vi "PatternRecognition.vi"() -> ()   [LabVIEW 2021]
uses:
  <vilib>/Analysis/baseanly.llb/Normalize Matrix.vi
  <vilib>/numeric/Random Number (Range) I64.vi
  <vilib>/Analysis/baseanly.llb/Real A x B.vi
  <vilib>/numeric/sub_Random U32.vi
  <vilib>/Analysis/Matrix/Numeric/Conversions/Matrix To Array - RM.vi
  <vilib>/Analysis/NI_AALBase.lvlib
  <vilib>/Analysis/Matrix/NI_Matrix.lvlib
  <vilib>/vision/NI_Vision_Development_Module.lvlib
panel:
  out "Confidence":dbl
  out "Pattern":dbl
  out "min value":dbl
  out "max value":dbl
  out "Elapsed Time Text":string
  out "Image":T1(plugin-control)
  in  "Init - Random":bool
  in  "index":i32
  in  "Paths":path[](array[path])
  out "Image Pixels":sgl[][](array[numeric])
  in  "Output":i32=1
  in  "2th layer":i32=2
  in  "1th layer":i32=3
  in  "Predict":bool
  out "Error":dbl[](array[numeric])
  in  "W1":dbl[][](array[numeric])
  out "Y":dbl[][](array[numeric])
  in  "Learn?":bool
  in  "Lr":dbl
  in  "stop":bool
  in  "Y_ideal":dbl[][][](array[numeric])
  in  "Bias 2":dbl[][](array[numeric]) format="%#_13g"
  in  "Bias 3":dbl[][](array[numeric]) format="%#_13g"
  in  "Bias 1":dbl[][](array[numeric]) format="%#_13g"
  in  "W2":dbl[][](array[numeric])
  in  "W3":dbl[][](array[numeric])
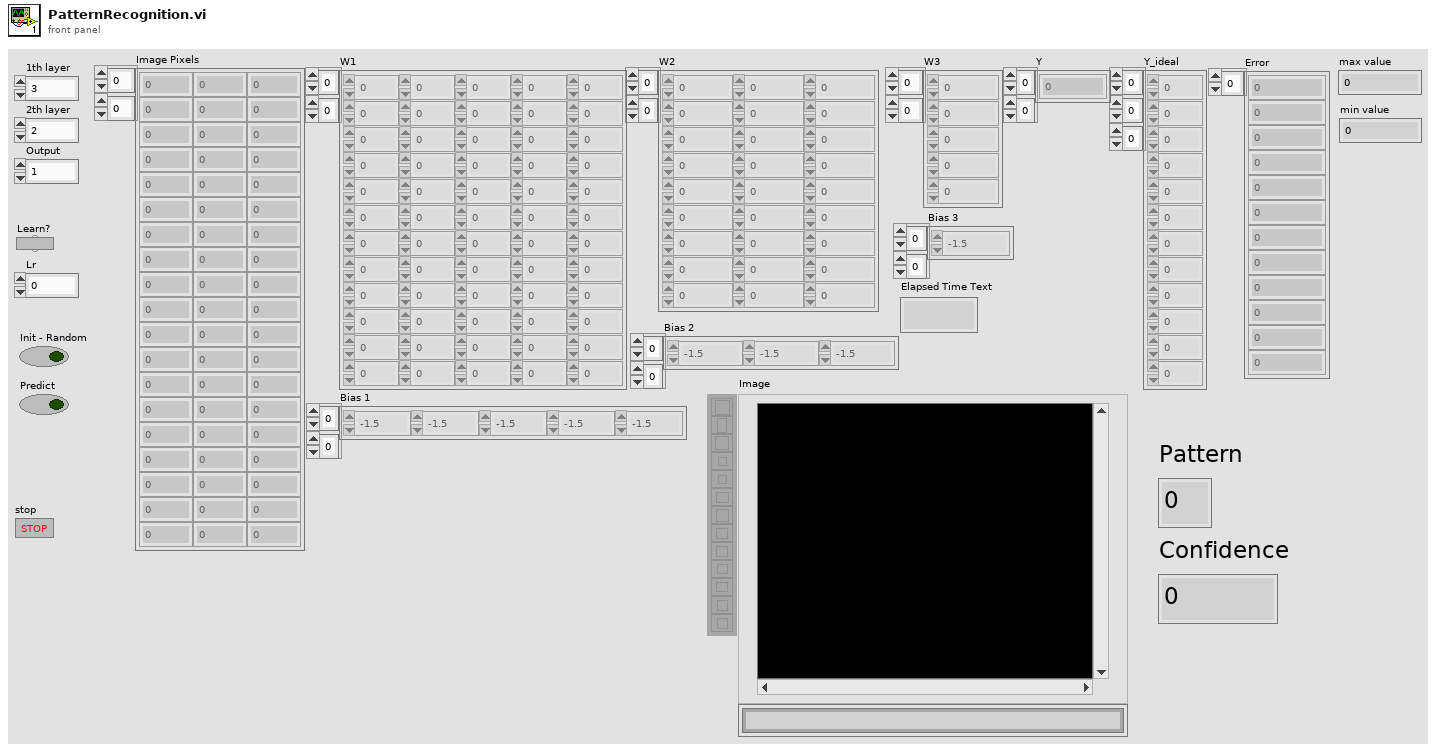
[diagram p1: front panel]
types:
  T1 = typedef "IMAQ Image.ctl" = refnum<image>
  T2 = typedef "Image Type" = u32
  T3 = typedef "NI_Matrix.lvlib/RealMatrix.ctl" = dbl[][]
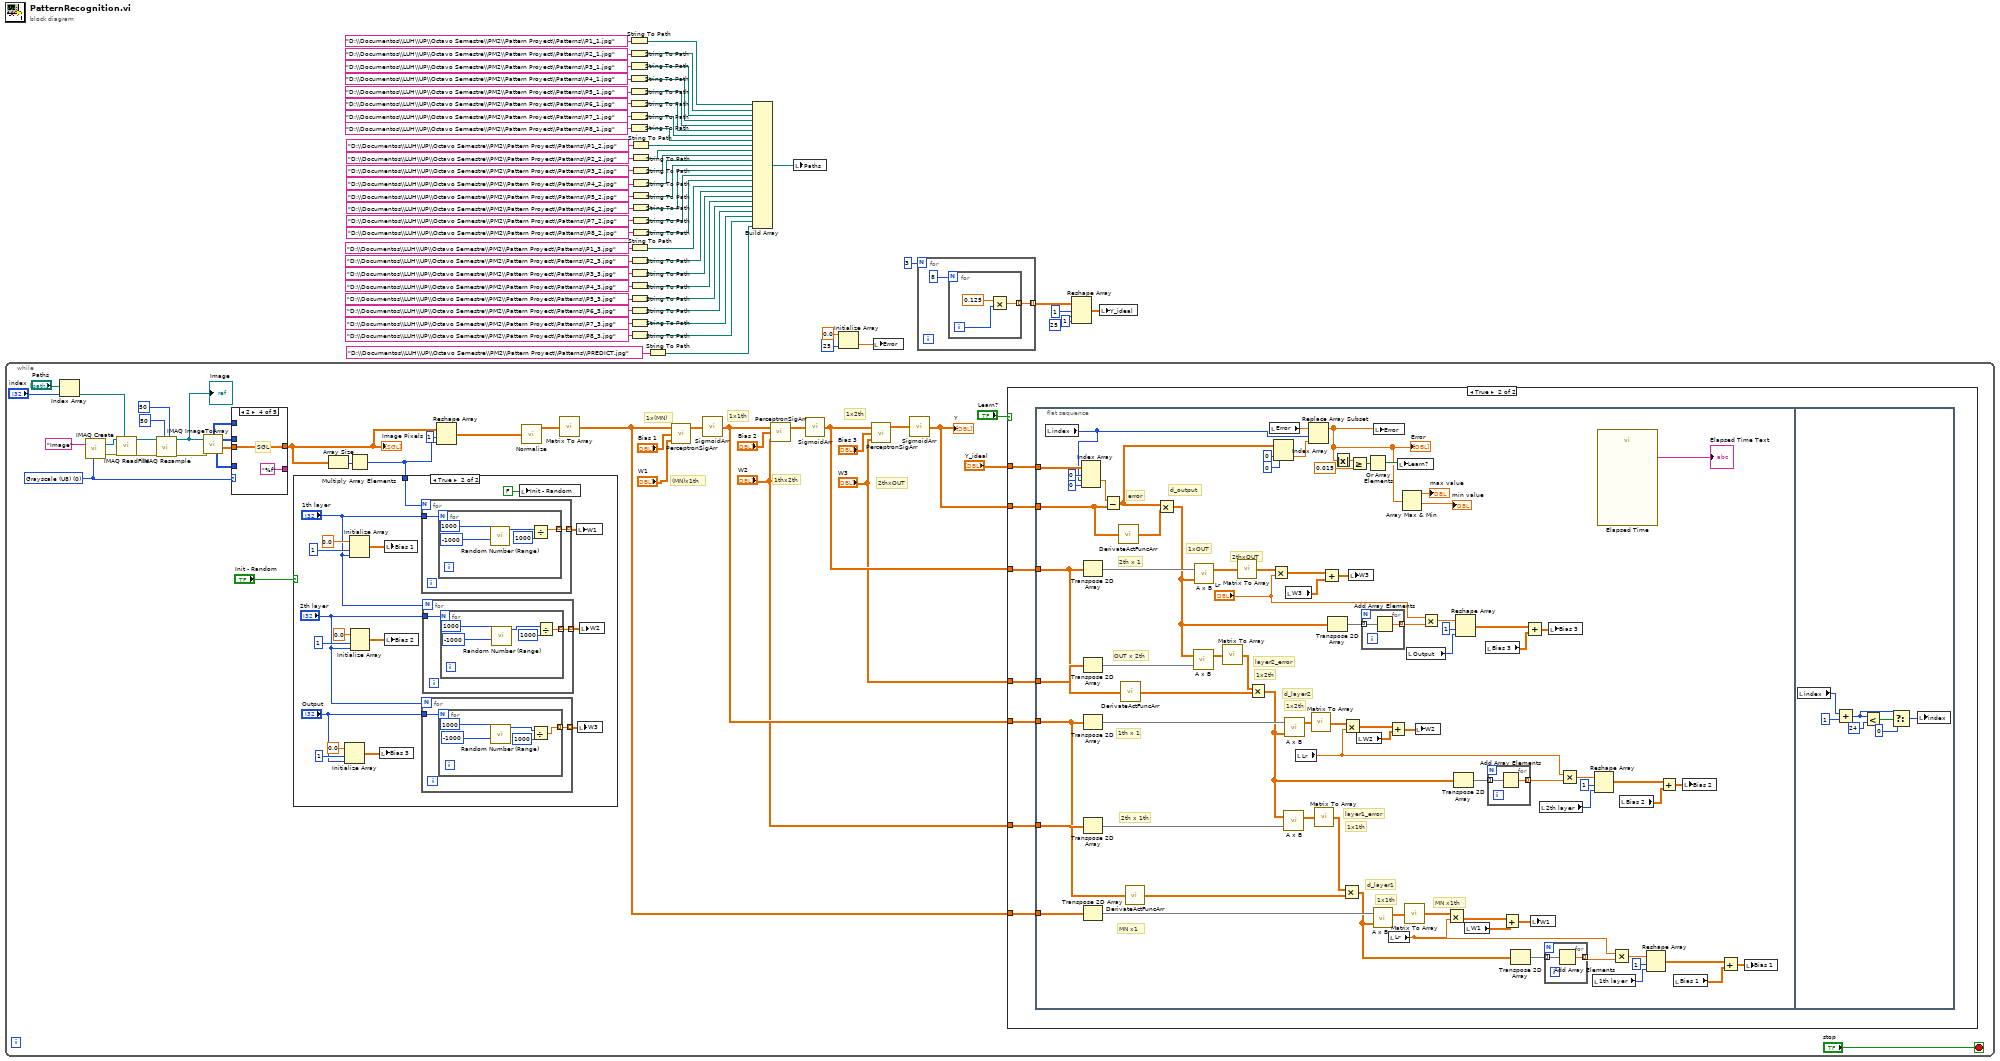
[diagram p0: block diagram]
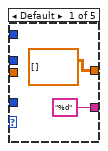
[diagram p3: hidden frame]
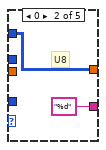
[diagram p4: hidden frame]
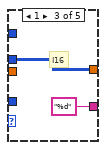
[diagram p5: hidden frame]
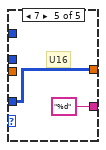
[diagram p6: hidden frame]
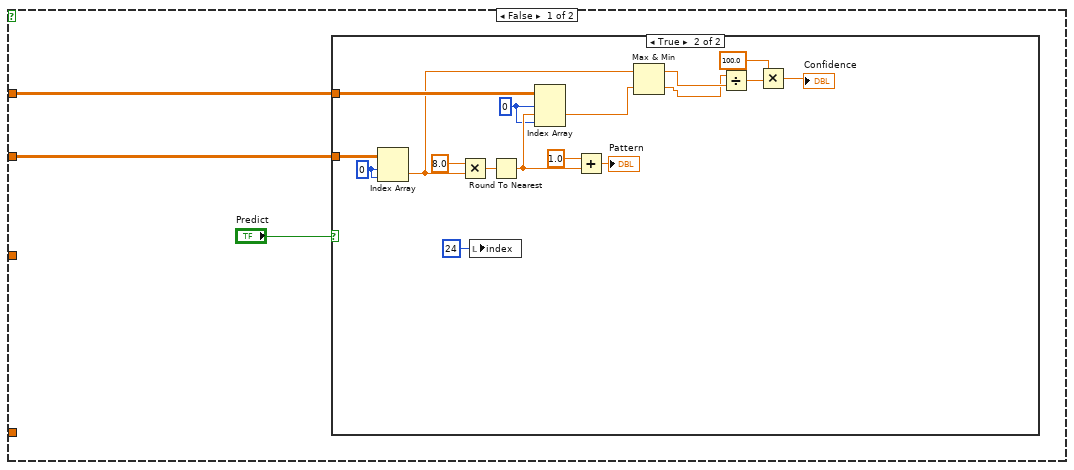
[diagram p7: hidden frame]
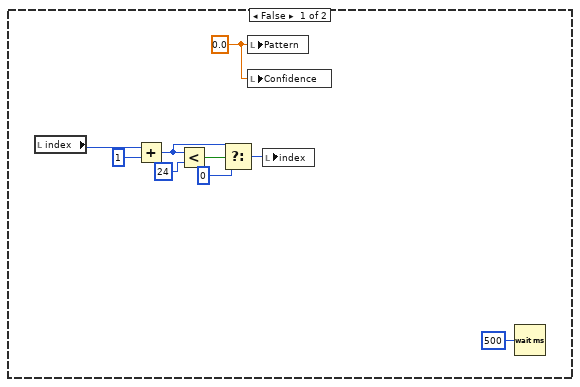
[diagram p8: hidden frame]
diagram:
  n1 = while {
    stop <- "stop" stop-if-true
    w82 = T2 0 items=["Grayscale (U8)", "Grayscale (I16)", "Grayscale (SGL)", "Complex (CSG)", "RGB (U32)", "HSL (U32)", "RGB (U64)", "Grayscale (U16)"] ("Image Type")
    # "2thxOUT"
    # "1x2th"
    # "1thx2th"
    # "1x1th"
    # "1x(MN)"
    # "(MN)x1th"
    n2 = Index Array(array="Paths", index="index") -> (element=w78:path)
    n3 = call "IMAQ Create"("Image Name"="Image", "Image Type"=w82) -> ("New Image"=w84:T1, "error out"=w85:errorcluster)  [unwired: 3 in]
    n4 = call "IMAQ ReadFile"("File Path"=w78, "error in (no error)"=w85, "Image"=w84) -> ("error out"=w72:errorcluster, "Image Out"=w65:T1)  [unwired: 4 in, 3 out]
    n5 = call "IMAQ Resample"("X Resolution"=50, "Y Resolution"=50, "error in (no error)"=w72, "Image Src"=w65) -> ("error out"=w71:errorcluster, "Image Dst Out"=w61:T1)  [unwired: 6 in]
    "Image" <- w61
    n6 = call "IMAQ ImageToArray"("error in (no error)"=w71, "Image"=w61) -> ("Image Pixels (U16)"=w79:u16[][], "Image Pixels (Float)"=w80:sgl[][], "Image Pixels (U8)"=w81:u8[][], "Image Pixels (I16)"=w83:i16[][])  [unwired: 2 in, 1 out]
    n7 = case shown="2" w82 {
      tunnel: w83 -> [_ _ w143 _ _]
      tunnel: w81 -> [_ w142 _ _ _]
      tunnel: w80 -> [_ _ _ w145 _]
      tunnel: w79 -> [_ _ _ _ w147]
      tunnel: [sgl[][] [] ("Image Pixels (Float)") w142 w143 w145 w147] -> w68
      tunnel: ["%d" ("Format-String") "%d" ("Format-String") "%d" ("Format-String") "%f" ("Format-String") "%d" ("Format-String")] -> _
      frame Default {
      }
      frame 0 {
        # "U8"
      }
      frame 1 {
        # "I16"
      }
      frame 2 {
        # "SGL"
      }
      frame 7 {
        # "U16"
      }
    }
    "Image Pixels" <- w68
    n8 = Array Size(array=w68) -> (size(s)=w74:i32[])
    n9 = Multiply Array Elements(1:w74) -> (0:w67:i32)
    n10 = case shown="True" "Init - Random" {
      tunnel: w67 -> [_ w116]
      frame False {
      }
      frame True {
        n11 = Initialize Array(0.0 ("element"), 1 ("dimension size"), "Output") -> (w101:dbl[][])
        n12 = Initialize Array(0.0 ("element"), 1 ("dimension size"), "1th layer") -> (w115:dbl[][])
        n13 = Initialize Array(0.0 ("element"), 1 ("dimension size"), "2th layer") -> (w110:dbl[][])
        n14 = local write "Bias 3"(w101) -> ()
        n15 = local write "Bias 1"(w115) -> ()
        n16 = local write "Bias 2"(w110) -> ()
        n17 = for {
          N: w116 -> [_]
          tunnel: "1th layer" -> [w133]
          tunnel: [w132] -> w112 mode=indexing
          n18 = for {
            N: w133 -> [_]
            tunnel: [w135] -> w132 mode=indexing
            n19 = call-poly <vilib>:"Random Number (Range).vi"("lower bound (-100)"=i64 -1000, "upper bound (100)"=i64 1000) -> ("number"=w136:i64)  [unwired: 9 in]
            n20 = Divide(x=w136, y=i64 1000) -> (x/y=w135:dbl)
          }
        }
        n21 = for {
          N: "2th layer" -> [_]
          tunnel: "Output" -> [w119]
          tunnel: [w118] -> w105 mode=indexing
          n22 = for {
            N: w119 -> [_]
            tunnel: [w120] -> w118 mode=indexing
            n23 = call-poly <vilib>:"Random Number (Range).vi"("lower bound (-100)"=i64 -1000, "upper bound (100)"=i64 1000) -> ("number"=w121:i64)  [unwired: 9 in]
            n24 = Divide(x=w121, y=i64 1000) -> (x/y=w120:dbl)
          }
        }
        n25 = for {
          N: "1th layer" -> [_]
          tunnel: "2th layer" -> [w126]
          tunnel: [w125] -> w106 mode=indexing
          n26 = for {
            N: w126 -> [_]
            tunnel: [w128] -> w125 mode=indexing
            n27 = call-poly <vilib>:"Random Number (Range).vi"("lower bound (-100)"=i64 -1000, "upper bound (100)"=i64 1000) -> ("number"=w127:i64)  [unwired: 9 in]
            n28 = Divide(x=w127, y=i64 1000) -> (x/y=w128:dbl)
          }
        }
        n29 = local write "Init - Random"(FALSE ("Init")) -> ()
        n30 = local write "W1"(w112) -> ()
        n31 = local write "W3"(w105) -> ()
        n32 = local write "W2"(w106) -> ()
      }
    }
    n33 = Reshape Array(w68, 1 ("dimension size"), w67) -> (w64:sgl[][])
    n34 = call-poly <vilib>:"Normalize.vi"("Matrix"=w64) -> ("Normalized Matrix"=w63:T3)  [unwired: 1 in, 3 out]
    n35 = call-poly <vilib>:"Matrix To Array.vi"("Real Matrix"=w63) -> ("Real 2D Array"=w62:dbl[][])
    n36 = call "PerceptronSigArr.vi"("Wa"="W1", "Bias"="Bias 1", "Xa"=w62) -> ("Y"=w94:dbl[][])
    n37 = call "SigmoidArr.vi"("x"=w94) -> ("Sigmoid"=w91:dbl[][])
    n38 = call "PerceptronSigArr.vi"("Wa"="W2", "Bias"="Bias 2", "Xa"=w91) -> ("Y"=w98:dbl[][])
    n39 = call "SigmoidArr.vi"("x"=w98) -> ("Sigmoid"=w89:dbl[][])
    n40 = call "PerceptronSigArr.vi"("Wa"="W3", "Bias"="Bias 3", "Xa"=w89) -> ("Y"=w96:dbl[][])
    n41 = call "SigmoidArr.vi"("x"=w96) -> ("Sigmoid"=w87:dbl[][])
    "Y" <- w87
    n42 = case shown="True" "Learn?" {
      tunnel: w87 -> [w150 w183]
      tunnel: "Y_ideal" -> [w149 w184]
      tunnel: w89 -> [_ w181]
      tunnel: "W3" -> [_ w182]
      tunnel: w91 -> [_ w179]
      tunnel: "W2" -> [_ w180]
      tunnel: w62 -> [_ w178]
      frame False {
        n43 = case shown="True" "Predict" {
          tunnel: w150 -> [_ w175]
          tunnel: w149 -> [_ w170]
          frame False {
            w152 = 0.0 ("Pattern")
            n44 = local read "index"() -> (w160:i32)
            n45 = Add(x=w160, y=1) -> (x+y=w156:i32)
            n46 = Less?(x=w156, y=24) -> (x < y?=w157:bool)
            n47 = Select(t=w156, s=w157, f=0) -> (s? t:f=w154:i32)
            n48 = local write "Pattern"(w152) -> ()
            n49 = local write "Confidence"(w152) -> ()
            n50 = local write "index"(w154) -> ()
            n51 = Wait (ms)(milliseconds to wait=u32 500) -> ()  [unwired: 1 out]
          }
          frame True {
            w168 = 0 ("disabled index (page)")
            w176 = 0 ("index (row)")
            n52 = Index Array(array=w175, index (row)=w176, index (col)=w176) -> (element=w164:dbl)
            n53 = Multiply(x=8.0, y=w164) -> (x*y=w171:dbl)
            n54 = local write "index"(24 ("index")) -> ()
            n55 = Round To Nearest(number=w171) -> (nearest integer value=w169:dbl)
            n56 = Index Array(array=w170, index (dim 0)=w168, index (dim 1)=w169, index (dim 2)=w168) -> (element=w163:dbl)
            n57 = Add(x=1.0, y=w169) -> (x+y=→"Pattern":dbl)
            n58 = Max & Min(x=w164, y=w163) -> (max(x,y)=w162:dbl, min(x,y)=w161:dbl)
            n59 = Divide(x=w161, y=w162) -> (x/y=w167:dbl)
            n60 = Multiply(x=100.0, y=w167) -> (x*y=→"Confidence":dbl)
          }
        }
      }
      frame True {
        n61 = flat-sequence {
          tunnel: w184 -> [w200]
          tunnel: w183 -> [w253]
          tunnel: w182 -> [w241]
          tunnel: w181 -> [w238]
          tunnel: w180 -> [w224]
          tunnel: w179 -> [w220]
          tunnel: w178 -> [w206]
          frame #0 {
            # "MN x1th"
            # "MN x1"
            # "1x1th"
            # "d_layer1"
            # "1x1th"
            # "layer1_error"
            # "2th x 1th"
            # "1th x 1"
            # "1x2th"
            # "OUT x 2th"
            # "d_layer2"
            # "1x2th"
            # "layer2_error"
            # "2thxOUT"
            # "1xOUT"
            # "2th x 1"
            # "d_output"
            # "error"
            n62 = local read "index"() -> (w196:i32)
            n63 = Index Array(array=w200, index (dim 0)=0 ("index (page)"), index (dim 1)=w196, index (dim 2)=0 ("disabled index (col)")) -> (element=w199:dbl)
            n64 = Transpose 2D Array(2D array=w238) -> (transposed array=w251:dbl[][])
            n65 = Transpose 2D Array(2D array=w241) -> (transposed array=w240:dbl[][])
            n66 = Transpose 2D Array(2D array=w220) -> (transposed array=w235:dbl[][])
            n67 = Transpose 2D Array(2D array=w224) -> (transposed array=w223:dbl[][])
            n68 = Transpose 2D Array(2D array=w206) -> (transposed array=w218:dbl[][])
            n69 = Subtract(x=w199, y=w253) -> (x-y=w191:dbl[][])
            n70 = call "DerivateActFuncArr.vi"("Input"=w253) -> ("Output"=w252:dbl[][])
            n71 = call "DerivateActFuncArr.vi"("Input"=w238) -> ("Output"=w239:dbl[][])
            n72 = call "DerivateActFuncArr.vi"("Input"=w220) -> ("Output"=w219:dbl[][])
            n73 = Multiply(x=w191, y=w252) -> (x*y=w205:dbl[][])
            n74 = call-poly <vilib>:"A x B.vi"("B"=w240, "A"=w205) -> ("A x B"=w237:T3)  [unwired: 1 out]
            n75 = call-poly <vilib>:"A x B.vi"("B"=w205, "A"=w251) -> ("A x B"=w250:T3)  [unwired: 1 out]
            n76 = call-poly <vilib>:"Matrix To Array.vi"("Real Matrix"=w237) -> ("Real 2D Array"=w236:dbl[][])
            n77 = call-poly <vilib>:"Matrix To Array.vi"("Real Matrix"=w250) -> ("Real 2D Array"=w249:dbl[][])
            n78 = Multiply ("Multiply.vi")(x=w236, y=w239) -> (x*y=w225:dbl[][])
            n79 = local read "Error"() -> (w204:dbl[])
            n80 = Multiply ("Multiply.vi")(x=w249, y="Lr") -> (x*y=w248:dbl[][])
            n81 = Index Array(array=w191, index (row)=0 ("index"), index (col)=0 ("disabled index (col)")) -> (element=w192:dbl)
            n82 = call-poly <vilib>:"A x B.vi"("B"=w223, "A"=w225) -> ("A x B"=w222:T3)  [unwired: 1 out]
            n83 = call-poly <vilib>:"A x B.vi"("B"=w225, "A"=w235) -> ("A x B"=w234:T3)  [unwired: 1 out]
            n84 = local read "W3"() -> (w263:dbl[][])
            n85 = local read "Lr"() -> (w194:dbl)
            n86 = Replace Array Subset(array=w204, new element=w192, index=w196) -> (w185:dbl[])
            "Error" <- w185
            n87 = call-poly <vilib>:"Matrix To Array.vi"("Real Matrix"=w234) -> ("Real 2D Array"=w233:dbl[][])
            n88 = call-poly <vilib>:"Matrix To Array.vi"("Real Matrix"=w222) -> ("Real 2D Array"=w221:dbl[][])
            n89 = Add ("Add.vi")(x=w248, y=w263) -> (x+y=w262:dbl[][])
            n90 = Transpose 2D Array(2D array=w205) -> (transposed array=w247:dbl[][])
            n91 = Absolute Value(x=w185) -> (abs(x)=w189:dbl[])
            n92 = Multiply ("Multiply.vi")(x=w221, y=w219) -> (x*y=w213:dbl[][])
            n93 = Multiply ("Multiply.vi")(x=w233, y=w194) -> (x*y=w232:dbl[][])
            n94 = local write "W3"(w262) -> ()
            n95 = Greater Or Equal?(x=w189, y=0.015 ("err")) -> (x >= y?=w202:bool[])
            n96 = local read "W2"() -> (w258:dbl[][])
            n97 = for {
              tunnel: w247 -> [w271] mode=indexing
              tunnel: [w270] -> w246 mode=indexing
              n98 = Add Array Elements(numeric array=w271) -> (sum=w270:dbl)
            }
            n99 = Or Array Elements(Boolean array=w202) -> (logical OR=w201:bool)
            n100 = call-poly <vilib>:"A x B.vi"("B"=w213, "A"=w218) -> ("A x B"=w217:T3)  [unwired: 1 out]
            n101 = local write "Error"(w185) -> ()
            n102 = Add ("Add.vi")(x=w232, y=w258) -> (x+y=w259:dbl[][])
            n103 = local read "Lr"() -> (w209:dbl)
            n104 = local write "Learn?"(w201) -> ()
            n105 = Array Max & Min(array=w185) -> (max value=→"max value":dbl, min value=→"min value":dbl)  [unwired: 2 out]
            n106 = call-poly <vilib>:"Matrix To Array.vi"("Real Matrix"=w217) -> ("Real 2D Array"=w216:dbl[][])
            n107 = local read "Output"() -> (w243:i32)
            n108 = local write "W2"(w259) -> ()
            n109 = Multiply ("Multiply.vi")(x="Lr", y=w246) -> (x*y=w245:dbl[])
            n110 = Multiply ("Multiply.vi")(x=w216, y=w209) -> (x*y=w215:dbl[][])
            n111 = Transpose 2D Array(2D array=w225) -> (transposed array=w231:dbl[][])
            n112 = Reshape Array(w245, 1 ("dimension size"), w243) -> (w242:dbl[][])
            n113 = local read "W1"() -> (w265:dbl[][])
            n114 = local read "Bias 3"() -> (w261:dbl[][])
            n115 = for {
              tunnel: w231 -> [w269] mode=indexing
              tunnel: [w268] -> w227 mode=indexing
              n116 = Add Array Elements(numeric array=w269) -> (sum=w268:dbl)
            }
            n117 = Add(x=w215, y=w265) -> (x+y=w264:dbl[][])
            n118 = Transpose 2D Array(2D array=w213) -> (transposed array=w214:dbl[][])
            n119 = Add(x=w242, y=w261) -> (x+y=w260:dbl[][])
            n120 = local write "W1"(w264) -> ()
            n121 = local read "2th layer"() -> (w228:i32)
            n122 = for {
              tunnel: w214 -> [w267] mode=indexing
              tunnel: [w266] -> w210 mode=indexing
              n123 = Add Array Elements(numeric array=w267) -> (sum=w266:dbl)
            }
            n124 = local write "Bias 3"(w260) -> ()
            n125 = Multiply ("Multiply.vi")(x=w194, y=w227) -> (x*y=w230:dbl[])
            n126 = local read "1th layer"() -> (w208:i32)
            n127 = Reshape Array(w230, 1 ("dimension size"), w228) -> (w226:dbl[][])
            n128 = call "Elapsed Time"() -> ("Elapsed Time Text"=→"Elapsed Time Text":string)  [unwired: 12 in, 7 out]
            n129 = Multiply ("Multiply.vi")(x=w209, y=w210) -> (x*y=w212:dbl[])
            n130 = local read "Bias 2"() -> (w257:dbl[][])
            n131 = Reshape Array(w212, 1 ("dimension size"), w208) -> (w207:dbl[][])
            n132 = Add(x=w226, y=w257) -> (x+y=w256:dbl[][])
            n133 = local read "Bias 1"() -> (w255:dbl[][])
            n134 = local write "Bias 2"(w256) -> ()
            n135 = Add(x=w207, y=w255) -> (x+y=w254:dbl[][])
            n136 = local write "Bias 1"(w254) -> ()
          }
          frame #1 {
            n137 = local read "index"() -> (w273:i32)
            n138 = Add(x=w273, y=1) -> (x+y=w275:i32)
            n139 = Less?(x=w275, y=24) -> (x < y?=w276:bool)
            n140 = Select(t=w275, s=w276, f=0) -> (s? t:f=w272:i32)
            n141 = local write "index"(w272) -> ()
          }
        }
      }
    }
  }
  n142 = String To Path(string="D:\\Documentos\\LUH\\UP\\Octavo Semestre\\PM2\\Pattern Proyect\\Patterns\\P1_1.jpg") -> (path=w30:path)
  n143 = String To Path(string="D:\\Documentos\\LUH\\UP\\Octavo Semestre\\PM2\\Pattern Proyect\\Patterns\\P2_1.jpg") -> (path=w29:path)
  n144 = String To Path(string="D:\\Documentos\\LUH\\UP\\Octavo Semestre\\PM2\\Pattern Proyect\\Patterns\\P3_1.jpg") -> (path=w28:path)
  n145 = String To Path(string="D:\\Documentos\\LUH\\UP\\Octavo Semestre\\PM2\\Pattern Proyect\\Patterns\\P4_1.jpg") -> (path=w27:path)
  n146 = String To Path(string="D:\\Documentos\\LUH\\UP\\Octavo Semestre\\PM2\\Pattern Proyect\\Patterns\\P5_1.jpg") -> (path=w26:path)
  n147 = String To Path(string="D:\\Documentos\\LUH\\UP\\Octavo Semestre\\PM2\\Pattern Proyect\\Patterns\\P6_1.jpg") -> (path=w25:path)
  n148 = String To Path(string="D:\\Documentos\\LUH\\UP\\Octavo Semestre\\PM2\\Pattern Proyect\\Patterns\\P7_1.jpg") -> (path=w24:path)
  n149 = String To Path(string="D:\\Documentos\\LUH\\UP\\Octavo Semestre\\PM2\\Pattern Proyect\\Patterns\\P8_1.jpg") -> (path=w23:path)
  n150 = String To Path(string="D:\\Documentos\\LUH\\UP\\Octavo Semestre\\PM2\\Pattern Proyect\\Patterns\\P1_3.jpg") -> (path=w14:path)
  n151 = String To Path(string="D:\\Documentos\\LUH\\UP\\Octavo Semestre\\PM2\\Pattern Proyect\\Patterns\\P2_3.jpg") -> (path=w13:path)
  n152 = String To Path(string="D:\\Documentos\\LUH\\UP\\Octavo Semestre\\PM2\\Pattern Proyect\\Patterns\\P3_3.jpg") -> (path=w12:path)
  n153 = String To Path(string="D:\\Documentos\\LUH\\UP\\Octavo Semestre\\PM2\\Pattern Proyect\\Patterns\\P4_3.jpg") -> (path=w11:path)
  n154 = String To Path(string="D:\\Documentos\\LUH\\UP\\Octavo Semestre\\PM2\\Pattern Proyect\\Patterns\\P5_3.jpg") -> (path=w10:path)
  n155 = String To Path(string="D:\\Documentos\\LUH\\UP\\Octavo Semestre\\PM2\\Pattern Proyect\\Patterns\\P6_3.jpg") -> (path=w9:path)
  n156 = String To Path(string="D:\\Documentos\\LUH\\UP\\Octavo Semestre\\PM2\\Pattern Proyect\\Patterns\\P7_3.jpg") -> (path=w8:path)
  n157 = String To Path(string="D:\\Documentos\\LUH\\UP\\Octavo Semestre\\PM2\\Pattern Proyect\\Patterns\\P8_3.jpg") -> (path=w7:path)
  n158 = String To Path(string="D:\\Documentos\\LUH\\UP\\Octavo Semestre\\PM2\\Pattern Proyect\\Patterns\\P1_2.jpg") -> (path=w22:path)
  n159 = String To Path(string="D:\\Documentos\\LUH\\UP\\Octavo Semestre\\PM2\\Pattern Proyect\\Patterns\\P2_2.jpg") -> (path=w21:path)
  n160 = String To Path(string="D:\\Documentos\\LUH\\UP\\Octavo Semestre\\PM2\\Pattern Proyect\\Patterns\\P3_2.jpg") -> (path=w20:path)
  n161 = String To Path(string="D:\\Documentos\\LUH\\UP\\Octavo Semestre\\PM2\\Pattern Proyect\\Patterns\\P4_2.jpg") -> (path=w19:path)
  n162 = String To Path(string="D:\\Documentos\\LUH\\UP\\Octavo Semestre\\PM2\\Pattern Proyect\\Patterns\\P5_2.jpg") -> (path=w18:path)
  n163 = String To Path(string="D:\\Documentos\\LUH\\UP\\Octavo Semestre\\PM2\\Pattern Proyect\\Patterns\\P6_2.jpg") -> (path=w17:path)
  n164 = String To Path(string="D:\\Documentos\\LUH\\UP\\Octavo Semestre\\PM2\\Pattern Proyect\\Patterns\\P7_2.jpg") -> (path=w16:path)
  n165 = String To Path(string="D:\\Documentos\\LUH\\UP\\Octavo Semestre\\PM2\\Pattern Proyect\\Patterns\\P8_2.jpg") -> (path=w15:path)
  n166 = String To Path(string="D:\\Documentos\\LUH\\UP\\Octavo Semestre\\PM2\\Pattern Proyect\\Patterns\\PREDICT.jpg") -> (path=w4:path)
  n167 = Build Array(w30, w29, w28, w27, w26, w25, w24, w23, w22, w21, w20, w19, w18, w17, w16, w15, w14, w13, w12, w11, w10, w9, w8, w7, w4) -> (w1:path[])
  n168 = local write "Paths"(w1) -> ()
  n169 = Initialize Array(0.0 ("element"), 25 ("dimension size")) -> (w47:dbl[])
  n170 = local write "Error"(w47) -> ()
  n171 = for {
    N: 3 -> [_]
    tunnel: [w279] -> w3 mode=indexing
    n172 = for {
      N: 8 -> [_]
      tunnel: [w281] -> w279 mode=indexing
      i -> [w282]
      n173 = Multiply(x=0.125, y=w282) -> (x*y=w281:dbl)
    }
  }
  n174 = Reshape Array(w3, 1 ("dimension size"), 25 ("dimension size"), 1 ("dimension size")) -> (w2:dbl[][][])
  n175 = local write "Y_ideal"(w2) -> ()
